vi "read_target.vi"(0 "Listbox  Target":i32[](listbox), 2 "Item Names":string[](array[string])) -> (1 "Array":string[](array[string]))   [LabVIEW 2015]
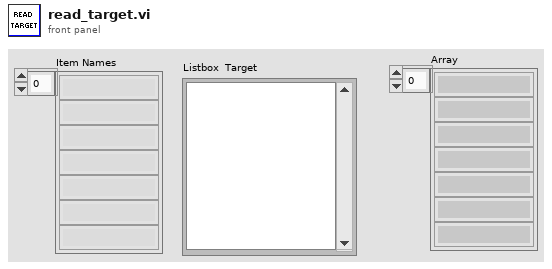
[diagram p1: front panel]
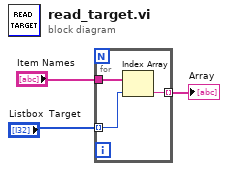
[diagram p0: block diagram]
diagram:
  n1 = for {
    tunnel: "Item Names" -> [w6]
    tunnel: "Listbox  Target" -> [w5] mode=indexing
    tunnel: [w4] -> w2 mode=indexing
    n2 = Index Array(array=w6, index=w5) -> (element=w4:string)
  }
  "Array" <- w2
